vi "score cube.vi"() -> ()   [LabVIEW 2018]
uses:
  <vilib>/myRIO/Instrument Drivers/Onboard IO/DIO/typedefs/DIO Reference.ctl
  <vilib>/myRIO/Common/Instrument Driver Framework/Utilities/typedefs/myRIO Generic Hardware Reference.ctl
  <vilib>/myRIO/Common/Instrument Driver Framework/Utilities/typedefs/Hardware Version Enum.ctl
  <vilib>/myRIO/Common/Instrument Driver Framework/Utilities/typedefs/myRIO v1.0 Reference.ctl
  <vilib>/myRIO/Common/Instrument Driver Framework/Utilities/typedefs/Generic FPGA Reference.ctl
  <vilib>/myRIO/Common/Instrument Driver Framework/myRIO v1.0/DIO/typedefs/DIO Channels List.ctl
  <vilib>/myRIO/Common/Instrument Driver Framework/myRIO v1.0/DIO/typedefs/DIO Channels Enum.ctl
  <vilib>/userdefined/High Color/nirio_resource_hc.ctl
  <vilib>/myRIO/Common/Instrument Driver Framework/Utilities/vis/Is FPGA Ref Available.vi
  <vilib>/myRIO/Common/Instrument Driver Framework/myRIO v1.0/DIO/vis/myRIO v1.1 Open DIO.vi
  <vilib>/myRIO/Instrument Drivers/Onboard IO/DIO/vis/Write.vi
  <vilib>/myRIO/Common/Instrument Driver Framework/Utilities/vis/Validate Channels.vi
  <vilib>/myRIO/Common/Instrument Driver Framework/myRIO v1.0/DIO/vis/myRIO v1.0 Reserve DIO.vi
  <vilib>/myRIO/Common/Instrument Driver Framework/myRIO v1.0/Resource Manager/vis/myRIO v1.0 Reserve Channel List.vi
  <vilib>/myRIO/Common/Instrument Driver Framework/myRIO v1.0/DIO/vis/myRIO v1.0 Build MUX Configuration DIO.vi
  <vilib>/myRIO/Common/Instrument Driver Framework/myRIO v1.0/Resource Manager/vis/myRIO v1.0 Reserve Channel.vi
  <vilib>/myRIO/Common/Instrument Driver Framework/myRIO v1.0/Resource Manager/vis/myRIO v1.0 Unreserve Channel.vi
  <vilib>/myRIO/Common/Instrument Driver Framework/myRIO v1.0/Resource Manager/vis/myRIO v1.0 Create Configuration List.vi
  <vilib>/myRIO/Common/Instrument Driver Framework/myRIO v1.0/Resource Manager/vis/myRIO v1.0 Build Mutex Name.vi
  <vilib>/Utility/VariantDataType/GetNumericInfo.vi
  <vilib>/Utility/error.llb/Error Cluster From Error Code.vi
  <vilib>/myRIO/Common/Instrument Driver Framework/myRIO v1.0/myRIO v1.1 Open.vi
  <vilib>/myRIO/Common/Instrument Driver Framework/Utilities/vis/IO Manager.vi
  <vilib>/myRIO/Common/Instrument Driver Framework/Utilities/vis/Configuration Manager.vi
  <vilib>/myRIO/Common/Instrument Driver Framework/myRIO v1.0/Resource Manager/vis/myRIO v1.0 Configure IO.vi
  <vilib>/myRIO/Common/Instrument Driver Framework/myRIO v1.0/myRIO v1.0 Close.vi
  <vilib>/myRIO/Common/Instrument Driver Framework/myRIO v1.0/DIO/vis/myRIO v1.0 Write DIO.vi
  <vilib>/myRIO/Express VI/Onboard Devices/LED/LED Express VI.xnode
  <vilib>/myRIO/Instrument Drivers/Onboard IO/DIO/vis/myRIO DIO Open.xnode
  <vilib>/myRIO/Instrument Drivers/Onboard IO/DIO/DIO.lvlib
  <vilib>/myRIO/Instrument Drivers/Onboard IO/DIO/vis/Read.vi
  <vilib>/myRIO/Express VI/Onboard Devices/Button/Button Express VI.xnode
  <vilib>/myRIO/Express VI/Onboard IO/DI/DI Express VI.xnode
panel:
  out "Boolean":bool
  out "Value":bool
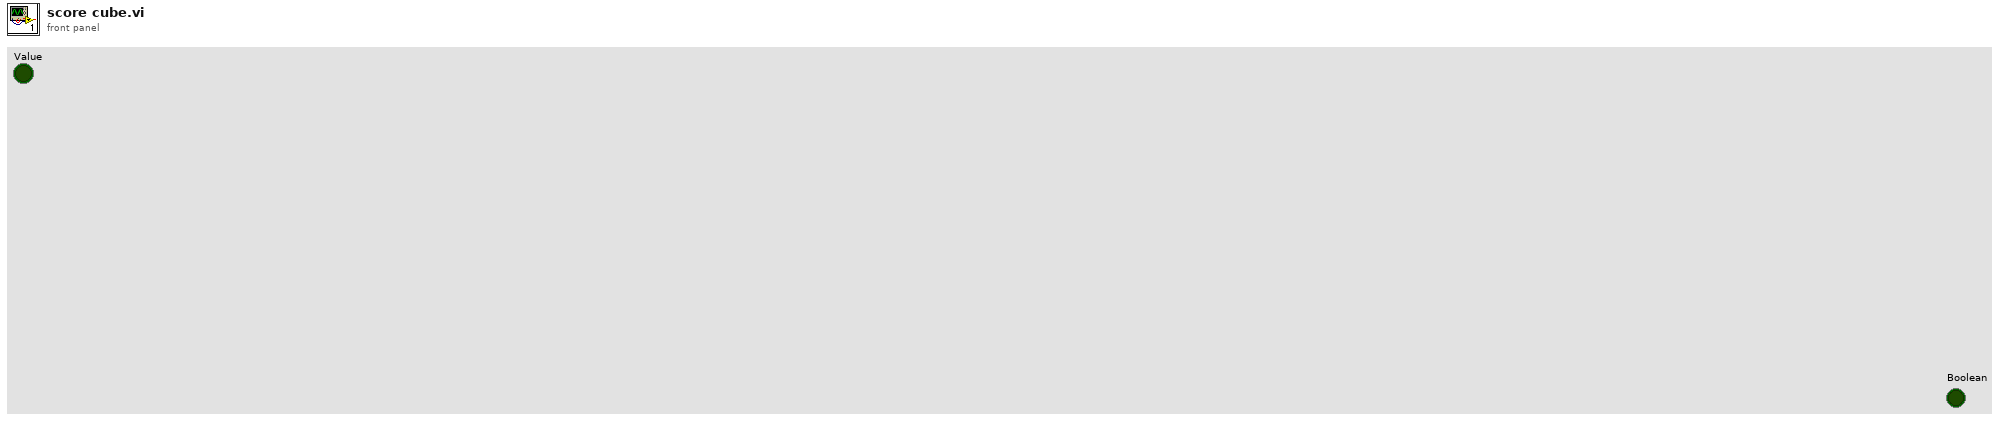
[diagram p1: front panel]
types:
  T1 = typedef "DIO.lvlib/DIO Reference.ctl" = cluster{"myRIO Reference":T2, "DIO Channels List":T6}
  T2 = typedef "myRIO Generic Hardware Reference.ctl" = cluster{"myRIO Model":T3, "myRIO Hardware Reference":T4}
  T3 = typedef "Hardware Version Enum.ctl" = enum16{"Unknown", "myRIO-1900", "myRIO-1950", "roboRIO", "NI ELVIS RIO CM", "ELVIS III"}
  T4 = typedef "myRIO v1.0 Reference.ctl" = cluster{"Generic FPGA Reference":T5, "Allow multiple opens":bool}
  T5 = typedef "Generic FPGA Reference.ctl" = refnum<k20>
  T6 = typedef "DIO Channels List.ctl" = T7[]
  T7 = typedef "DIO Channels Enum.ctl" = enum16{"Not Connected", "C/DIO0", "C/DIO1", "C/DIO2", "C/DIO3", "C/DIO4", "C/DIO5", "C/DIO6", "C/DIO7", "A/DIO0", "A/DIO1", "A/DIO2", "A/DIO3", "A/DIO4", "A/DIO5", "A/DIO6", "A/DIO7", "A/DIO8", "A/DIO9", "A/DIO10", "A/DIO11", "A/DIO12", "A/DIO13", "A/DIO14", "A/DIO15", "A/DIO16", "A/DIO17", "A/DIO18", "A/DIO19", "B/DIO0", "B/DIO1", "B/DIO2", "B/DIO3", "B/DIO4", "B/DIO5", "B/DIO6", "B/DIO7", "B/DIO8", "B/DIO9", "B/DIO10", "B/DIO11", "B/DIO12", "B/DIO13", "B/DIO14", "B/DIO15", "B/DIO16", "B/DIO17", "B/DIO18", "B/DIO19", "LED0", "LED1", "LED2", "LED3", "Button0", "DIO/DIO0", "DIO/DIO1", "DIO/DIO2", "DIO/DIO3", "DIO/DIO4", "DIO/DIO5", "DIO/DIO6", "DIO/DIO7", "DIO/DIO8", "DIO/DIO9", "SPI/CS0", "SPI/CS1", "SPI/CS2", "SPI/CS3", "LED RADIO (Green)", "LED RADIO (Red)", "LED COMM (Green)", "LED COMM (Red)", "LED MODE (Green)", "LED MODE (Red)"}
  T8 = typedef "nirio_resource_hc.ctl" = tag
  T9 = enum16{"shoulder", "elbow", "wrist", "base", "gripper"}
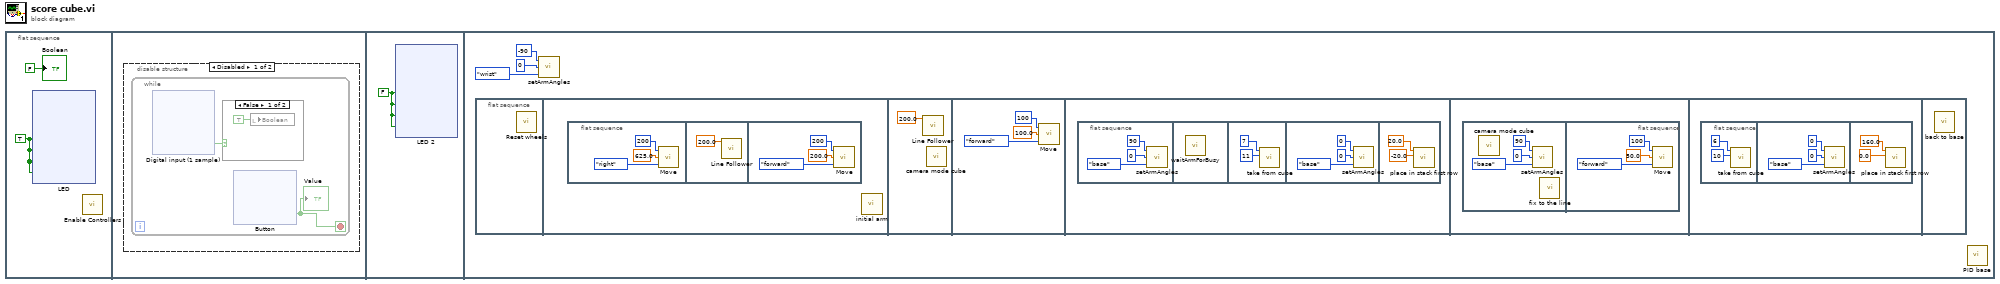
[diagram p0: block diagram]
diagram:
  n1 = flat-sequence {
    frame #0 {
      w2 = TRUE ("LED0")
      n2 = xnode "LED"("LED0"=w2, "LED1"=w2, "LED2"=w2, "LED3"=w2) -> ()  [unwired: 1 in, 1 out]
      n3 = call "Enable Controllers.vi"() -> ()  [unwired: 12 in]
      "Boolean" <- FALSE ("Boolean")
    }
    frame #1 {
      n4 = disable-structure shown="Disabled" {
        frame Disabled {
          n5 = while {
            stop <- w42 stop-if-true
            n6 = xnode "Digital input (1 sample)"() -> ("A/DIO0 (Pin 11)"=w41:bool)  [unwired: 1 in, 1 out]
            n7 = case shown="False" w41 {
              frame False {
                n8 = local write "Boolean"(TRUE ("Boolean")) -> ()
              }
              frame True {
              }
            }
            n9 = xnode "Button"() -> ("Value"=w42:bool)  [unwired: 1 in, 1 out]
            "Value" <- w42
          }
        }
        frame Enabled {
        }
      }
    }
    frame #2 {
      w114 = FALSE ("LED0")
      n10 = xnode "LED 2"("LED0"=w114, "LED1"=w114, "LED2"=w114, "LED3"=w114) -> ()  [unwired: 1 in, 1 out]
    }
    frame #3 {
      n11 = flat-sequence {
        frame #0 {
          n12 = call "Reset wheels.vi"() -> ()  [unwired: 12 in]
        }
        frame #1 {
          n13 = flat-sequence {
            frame #0 {
              n14 = call "Move.vi"("Enum"=enum16{"forward", "backward", "left", "right"}."right", "distance"=625.0, "speed"=200) -> ()  [unwired: 1 in]
            }
            frame #1 {
              n15 = call "Line Follower.vi"("speed"=200.0) -> ()  [unwired: 11 in]
            }
            frame #2 {
              n16 = call "Move.vi"("Enum"=enum16{"forward", "backward", "left", "right"}."forward", "distance"=200.0, "speed"=200) -> ()  [unwired: 1 in]
            }
          }
          n17 = call "initial arm.vi"() -> ()  [unwired: 12 in]
        }
        frame #2 {
          n18 = call "Line Follower.vi"("speed"=200.0) -> ()  [unwired: 11 in]
          n19 = call "camera mode cube.vi"() -> ()  [unwired: 12 in]
        }
        frame #3 {
          n20 = call "Move.vi"("Enum"=enum16{"forward", "backward", "left", "right"}."forward", "distance"=100.0, "speed"=100) -> ()  [unwired: 1 in]
        }
        frame #4 {
          n21 = flat-sequence {
            frame #0 {
              n22 = call "setArmAngles.vi"("Enum"=T9."base", "speed"=0, "angle"=90) -> ()  [unwired: 1 in]
            }
            frame #1 {
              n23 = call "waitArmForBusy.vi"() -> ()  [unwired: 12 in]
            }
            frame #2 {
              n24 = call "take from cube.vi"("c2"=11, "c1"=7) -> ()  [unwired: 10 in]
            }
            frame #3 {
              n25 = call "setArmAngles.vi"("Enum"=T9."base", "speed"=0, "angle"=0) -> ()  [unwired: 1 in]
            }
            frame #4 {
              n26 = call "place in stack first row.vi"("c2"=-20.0, "c1"=20.0) -> ()  [unwired: 10 in]
            }
          }
        }
        frame #5 {
          n27 = flat-sequence {
            frame #0 {
              n28 = call "camera mode cube.vi"() -> ()  [unwired: 12 in]
              n29 = call "setArmAngles.vi"("Enum"=T9."base", "speed"=0, "angle"=90) -> ()  [unwired: 1 in]
              n30 = call "fix to the line.vi"() -> ()  [unwired: 12 in]
            }
            frame #1 {
              n31 = call "Move.vi"("Enum"=enum16{"forward", "backward", "left", "right"}."forward", "distance"=50.0, "speed"=100) -> ()  [unwired: 1 in]
            }
          }
        }
        frame #6 {
          n32 = flat-sequence {
            frame #0 {
              n33 = call "take from cube.vi"("c2"=10, "c1"=6) -> ()  [unwired: 10 in]
            }
            frame #1 {
              n34 = call "setArmAngles.vi"("Enum"=T9."base", "speed"=0, "angle"=0) -> ()  [unwired: 1 in]
            }
            frame #2 {
              n35 = call "place in stack first row.vi"("c2"=0.0, "c1"=160.0) -> ()  [unwired: 10 in]
            }
          }
        }
        frame #7 {
          n36 = call "back to base.vi"() -> ()  [unwired: 12 in]
        }
      }
      n37 = call "setArmAngles.vi"("Enum"=T9."wrist", "speed"=0, "angle"=-90) -> ()  [unwired: 1 in]
      n38 = call "PID base.vi"() -> ()  [unwired: 12 in]
    }
  }
